vi "reward_behavior_michelle_visjitter_conswinAdapt_enticefx_TSLog_VF_fortraining_lightdetectionV2.vi"() -> ()   [LabVIEW 2019]
doc: "The myRIO Project template acquires acceleration data from the onboard accelerometer and displays the changes of acceleration values in a waveform chart."
uses:
  <vilib>/Analysis/Matrix/Datatypes/RealMatrix.ctl
  <vilib>/Utility/miscctls.llb/LVDateTimeRec.ctl
  <vilib>/myRIO/Instrument Drivers/Onboard IO/DIO/typedefs/DIO Reference.ctl
  <vilib>/myRIO/Common/Instrument Driver Framework/Utilities/typedefs/myRIO Generic Hardware Reference.ctl
  <vilib>/myRIO/Common/Instrument Driver Framework/Utilities/typedefs/Hardware Version Enum.ctl
  <vilib>/myRIO/Common/Instrument Driver Framework/Utilities/typedefs/myRIO v1.0 Reference.ctl
  <vilib>/myRIO/Common/Instrument Driver Framework/Utilities/typedefs/Generic FPGA Reference.ctl
  <vilib>/myRIO/Common/Instrument Driver Framework/myRIO v1.0/DIO/typedefs/DIO Channels List.ctl
  <vilib>/myRIO/Common/Instrument Driver Framework/myRIO v1.0/DIO/typedefs/DIO Channels Enum.ctl
  <vilib>/userdefined/High Color/nirio_resource_hc.ctl
  <vilib>/myRIO/Common/Instrument Driver Framework/myRIO v1.0/Encoder/typedefs/Encoder Signal Mode.ctl
  <vilib>/myRIO/Instrument Drivers/Onboard IO/Encoder/typedefs/Encoder Reference.ctl
  <vilib>/myRIO/Common/Instrument Driver Framework/myRIO v1.0/Encoder/typedefs/Encoder Channels Enum.ctl
  <vilib>/myRIO/Common/Instrument Driver Framework/myRIO v1.0/Encoder/typedefs/Encoder Configuration v1.0.ctl
  <vilib>/myRIO/Instrument Drivers/Onboard IO/AI/typedefs/AI Reference.ctl
  <vilib>/myRIO/Common/Instrument Driver Framework/myRIO v1.0/AI/typedefs/AI Channels List.ctl
  <vilib>/myRIO/Common/Instrument Driver Framework/myRIO v1.0/AI/typedefs/AI Channels Enum.ctl
  <vilib>/myRIO/Common/Instrument Driver Framework/Utilities/typedefs/Analog Scaling Constants List.ctl
  <vilib>/myRIO/Common/Instrument Driver Framework/Utilities/typedefs/Analog Scaling Constants.ctl
  <vilib>/myRIO/Instrument Drivers/Onboard IO/AO/typedefs/AO Reference.ctl
  <vilib>/myRIO/Common/Instrument Driver Framework/myRIO v1.0/AO/typedefs/AO Channels List.ctl
  <vilib>/myRIO/Common/Instrument Driver Framework/myRIO v1.0/AO/typedefs/AO Channels Enum.ctl
  <vilib>/myRIO/Common/Instrument Driver Framework/Utilities/vis/Is FPGA Ref Available.vi
  <vilib>/myRIO/Common/Instrument Driver Framework/myRIO v1.0/DIO/vis/myRIO v1.1 Open DIO.vi
  <vilib>/myRIO/Instrument Drivers/Onboard IO/DIO/vis/Write.vi
  <vilib>/myRIO/Common/Instrument Driver Framework/myRIO v1.0/Encoder/vis/myRIO v1.1 Open Encoder.vi
  <vilib>/myRIO/Instrument Drivers/Onboard IO/Encoder/vis/Read.vi
  <vilib>/myRIO/Common/Instrument Driver Framework/myRIO v1.0/AI/vis/myRIO v1.1 Open AI.vi
  <vilib>/myRIO/Instrument Drivers/Onboard IO/AI/vis/Read.vi
  <vilib>/myRIO/Common/Instrument Driver Framework/myRIO v1.0/AO/vis/myRIO v1.1 Open AO.vi
  <vilib>/myRIO/Instrument Drivers/Onboard IO/AO/vis/Write.vi
  <vilib>/myRIO/Instrument Drivers/Onboard IO/DIO/vis/Read.vi
  <vilib>/myRIO/Common/Instrument Driver Framework/Utilities/vis/Validate Channels.vi
  <vilib>/myRIO/Common/Instrument Driver Framework/myRIO v1.0/DIO/vis/myRIO v1.0 Reserve DIO.vi
  <vilib>/myRIO/Common/Instrument Driver Framework/myRIO v1.0/Encoder/vis/myRIO v1.0 Reserve Encoder.vi
  <vilib>/myRIO/Common/Instrument Driver Framework/myRIO v1.0/AI/vis/myRIO v1.0 Reserve AI.vi
  <vilib>/myRIO/Common/Instrument Driver Framework/myRIO v1.0/AO/vis/myRIO v1.0 Reserve AO.vi
  <vilib>/myRIO/Common/Instrument Driver Framework/myRIO v1.0/Resource Manager/vis/myRIO v1.0 Reserve Channel List.vi
  <vilib>/myRIO/Common/Instrument Driver Framework/myRIO v1.0/DIO/vis/myRIO v1.0 Build MUX Configuration DIO.vi
  <vilib>/myRIO/Common/Instrument Driver Framework/myRIO v1.0/Encoder/vis/myRIO v1.0 Build MUX Configuration Encoder.vi
  <vilib>/myRIO/Common/Instrument Driver Framework/myRIO v1.0/AI/vis/myRIO v1.0 Build MUX Configuration AI.vi
  <vilib>/myRIO/Common/Instrument Driver Framework/myRIO v1.0/AO/vis/myRIO v1.0 Build MUX Configuration AO.vi
  <vilib>/myRIO/Common/Instrument Driver Framework/myRIO v1.0/Resource Manager/vis/myRIO v1.0 Reserve Channel.vi
  <vilib>/myRIO/Common/Instrument Driver Framework/myRIO v1.0/Resource Manager/vis/myRIO v1.0 Unreserve Channel.vi
  <vilib>/myRIO/Common/Instrument Driver Framework/myRIO v1.0/Resource Manager/vis/myRIO v1.0 Create Configuration List.vi
  <vilib>/myRIO/Common/Instrument Driver Framework/myRIO v1.0/Resource Manager/vis/myRIO v1.0 Build Mutex Name.vi
  <vilib>/Utility/VariantDataType/GetNumericInfo.vi
  <vilib>/Utility/error.llb/Error Cluster From Error Code.vi
  <vilib>/myRIO/Common/Instrument Driver Framework/myRIO v1.0/myRIO v1.1 Open.vi
  <vilib>/myRIO/Common/Instrument Driver Framework/Utilities/vis/IO Manager.vi
  <vilib>/myRIO/Common/Instrument Driver Framework/Utilities/vis/Configuration Manager.vi
  <vilib>/myRIO/Common/Instrument Driver Framework/myRIO v1.0/Resource Manager/vis/myRIO v1.0 Configure IO.vi
  <vilib>/myRIO/Common/Instrument Driver Framework/myRIO v1.0/myRIO v1.0 Close.vi
  <vilib>/myRIO/Common/Instrument Driver Framework/myRIO v1.0/Encoder/vis/myRIO v1.0 Configure Encoder.vi
  <vilib>/myRIO/Common/Instrument Driver Framework/myRIO v1.0/Encoder/vis/myRIO v1.0 Read Encoder.vi
  <vilib>/myRIO/Common/Instrument Driver Framework/myRIO v1.0/DIO/vis/myRIO v1.0 Write DIO.vi
  <vilib>/myRIO/Common/Instrument Driver Framework/myRIO v1.0/DIO/vis/myRIO v1.0 Read DIO.vi
  <vilib>/myRIO/Common/Instrument Driver Framework/myRIO v1.0/AI/vis/myRIO v1.0 Get Scaling Constants AI.vi
  <vilib>/myRIO/Common/Instrument Driver Framework/myRIO v1.0/AI/vis/myRIO v1.0 Read AI.vi
  <vilib>/myRIO/Common/Instrument Driver Framework/myRIO v1.0/AO/vis/myRIO v1.0 Get Scaling Constants AO.vi
  <vilib>/myRIO/Common/Instrument Driver Framework/myRIO v1.0/AO/vis/myRIO v1.0 Write AO.vi
  <vilib>/myRIO/Express VI/Onboard IO/Encoder/Encoder Express VI.xnode
  <vilib>/myRIO/Instrument Drivers/Onboard IO/Encoder/vis/myRIO Encoder Open.xnode
  <vilib>/myRIO/Common/Instrument Driver Framework/myRIO v1.0/Encoder/typedefs/Encoder Count Direction Enum.ctl
  <vilib>/myRIO/Express VI/Onboard IO/DO/DO Express VI.xnode
  <vilib>/myRIO/Instrument Drivers/Onboard IO/DIO/vis/myRIO DIO Open.xnode
  <vilib>/myRIO/Express VI/Onboard IO/DI/DI Express VI.xnode
  <vilib>/myRIO/Express VI/Onboard IO/AI/AI Express VI.xnode
  <vilib>/myRIO/Instrument Drivers/Onboard IO/AI/vis/myRIO AI Open.xnode
  <vilib>/myRIO/Express VI/Onboard IO/AO/AO Express VI.xnode
  <vilib>/myRIO/Instrument Drivers/Onboard IO/AO/vis/myRIO AO Open.xnode
  <vilib>/myRIO/Instrument Drivers/Onboard IO/Encoder/Encoder.lvlib
  <vilib>/myRIO/Instrument Drivers/Onboard IO/DIO/DIO.lvlib
  <vilib>/myRIO/Instrument Drivers/Onboard IO/AI/AI.lvlib
  <vilib>/myRIO/Instrument Drivers/Onboard IO/AO/AO.lvlib
  <vilib>/Analysis/Matrix/NI_Matrix.lvlib
panel:
  out "StartTime":dbl
  out "TimeStampTime":dbl
  out "initiatedlag":dbl
  out "NeedLag":bool=TRUE
  out "date time rec":T1
  out "InitiationLag":i32
  out "LightTrig":bool=TRUE
  out "LightAvg":dbl=0.15
  out "LimitCalc":dbl
  out "LightLimit":dbl
  out "LightTS":dbl[][](array[numeric])
  out "LightDerivPlot":dbl[](graph)
  out "LightDeriv":dbl
  out "LightOn":bool=TRUE
  out "Light":dbl
  out "Lightplot":dbl[](graph)
  out "LightArray":dbl[](array[numeric])
  out "AutoEnticeLimit":i32=1000
  out "GetVidFrame":i32
  out "VidTS":dbl[][](array[numeric])
  out "EntTS":dbl[][](array[numeric])
  out "TimeLag":dbl
  out "Lag2":dbl
  out "TestTime":dbl
  out "RewTS":dbl[][](array[numeric])
  out "ConsTS":dbl[][](array[numeric])
  out "LickTS":dbl[][](array[numeric])
  out "ContrastChoice":dbl
  out "Its":i32
  out "BurstCriteria":dbl
  out "LickBurst 2":bool
  out "LickBurst":bool
  out "Enticements":i32
  in  "Entice":bool
  out "Misses":i32
  out "GoAhead":bool
  out "TimeOutDuration":i32
  out "ActiveTime":dbl
  out "ConsumptionGo":bool=TRUE
  out "Consumption_Period":i32
  out "Watch_Display":bool=TRUE
  in  "Give reward":bool
  out "Timings":dbl[](array[numeric])
  out "ISI":dbl
  out "ISI start time":dbl
  out "Time_out":bool=TRUE
  out "Time since lick":dbl
  out "Time of last lick":dbl
  out "Rewarded trials":dbl[](array[numeric])
  out "Rewards":u16
  out "Active Trial":bool
  out "Array temp2":T2
  out "Stimuli Loaded":bool
  out "Stim_ID":dbl[](array[numeric])
  out "Reward_mat":dbl[](array[numeric])
  out "Reward":bool=TRUE
  out "Frame clock":i32
  out "Licks":u32
  out "Lick":bool
  out "Time":dbl
  out "Stop":bool
  in  "Frames to collect":u32
  out "Overflow?":bool
  out "Counter Value":i32
  out "Velocity":dbl
  out "Velocity Plot":dbl[](graph)
  out "Velocity array":dbl[](array[numeric])
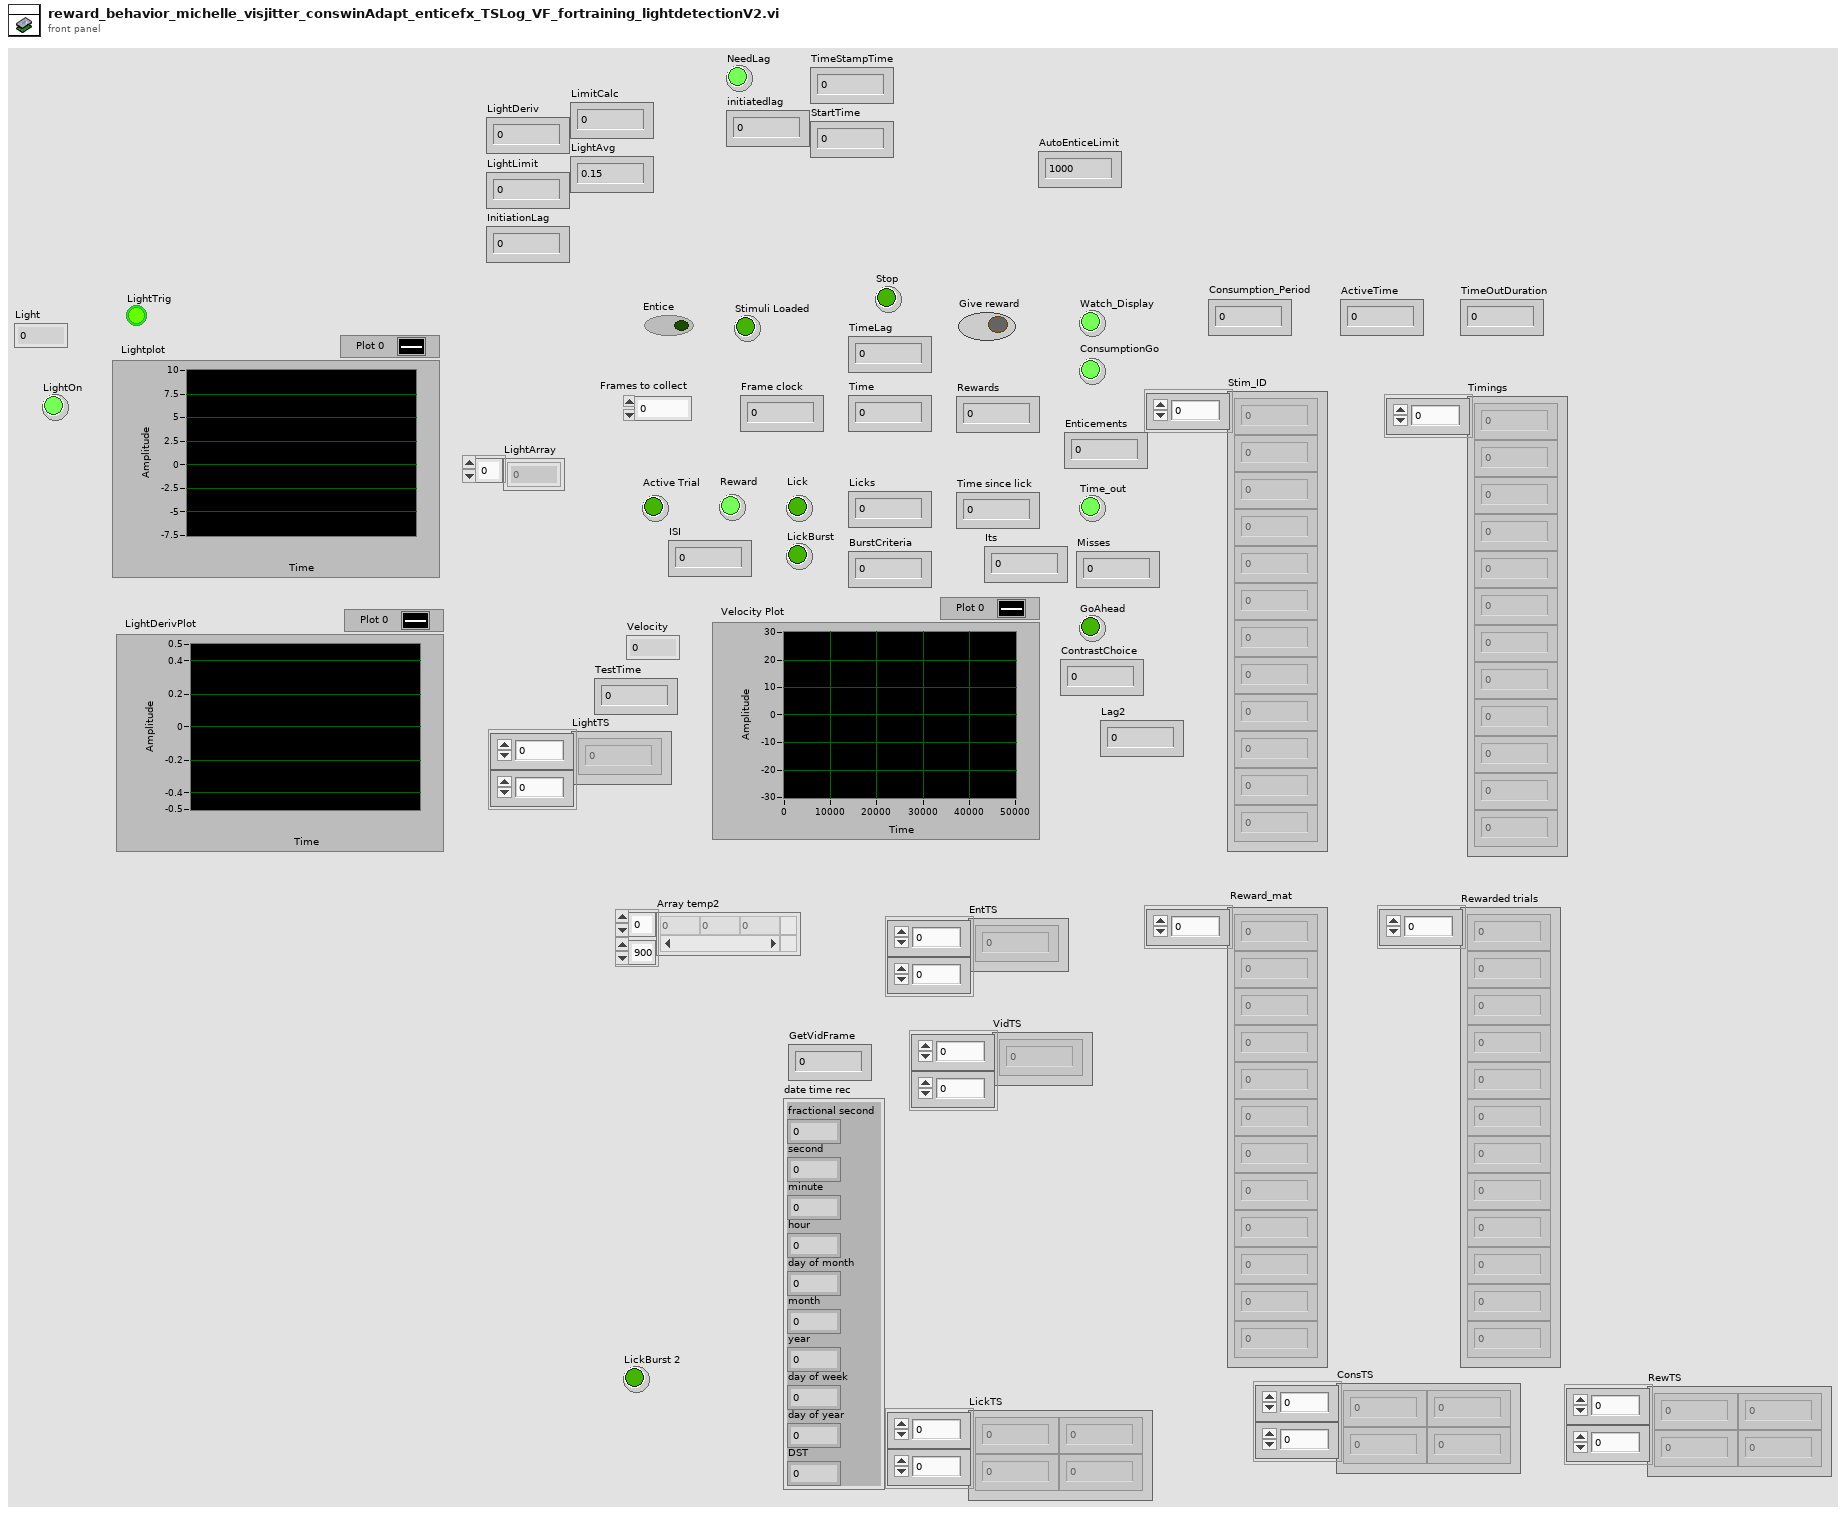
[diagram p1: front panel]
types:
  T1 = typedef "LVDateTimeRec.ctl" = cluster{"fractional second":dbl, "second":i32, "minute":i32, "hour":i32, "day of month":i32, "month":i32, "year":i32, "day of week":i32, "day of year":i32, "DST":i32}
  T2 = typedef "NI_Matrix.lvlib/RealMatrix.ctl" = dbl[][]
  T3 = typedef "DIO.lvlib/DIO Reference.ctl" = cluster{"myRIO Reference":T4, "DIO Channels List":T8}
  T4 = typedef "myRIO Generic Hardware Reference.ctl" = cluster{"myRIO Model":T5, "myRIO Hardware Reference":T6}
  T5 = typedef "Hardware Version Enum.ctl" = enum16{"Unknown", "myRIO-1900", "myRIO-1950", "roboRIO", "NI ELVIS RIO CM", "ELVIS III"}
  T6 = typedef "myRIO v1.0 Reference.ctl" = cluster{"Generic FPGA Reference":T7, "Allow multiple opens":bool}
  T7 = typedef "Generic FPGA Reference.ctl" = refnum<k20>
  T8 = typedef "DIO Channels List.ctl" = T9[]
  T9 = typedef "DIO Channels Enum.ctl" = enum16{"Not Connected", "C/DIO0", "C/DIO1", "C/DIO2", "C/DIO3", "C/DIO4", "C/DIO5", "C/DIO6", "C/DIO7", "A/DIO0", "A/DIO1", "A/DIO2", "A/DIO3", "A/DIO4", "A/DIO5", "A/DIO6", "A/DIO7", "A/DIO8", "A/DIO9", "A/DIO10", "A/DIO11", "A/DIO12", "A/DIO13", "A/DIO14", "A/DIO15", "A/DIO16", "A/DIO17", "A/DIO18", "A/DIO19", "B/DIO0", "B/DIO1", "B/DIO2", "B/DIO3", "B/DIO4", "B/DIO5", "B/DIO6", "B/DIO7", "B/DIO8", "B/DIO9", "B/DIO10", "B/DIO11", "B/DIO12", "B/DIO13", "B/DIO14", "B/DIO15", "B/DIO16", "B/DIO17", "B/DIO18", "B/DIO19", "LED0", "LED1", "LED2", "LED3", "Button0", "DIO/DIO0", "DIO/DIO1", "DIO/DIO2", "DIO/DIO3", "DIO/DIO4", "DIO/DIO5", "DIO/DIO6", "DIO/DIO7", "DIO/DIO8", "DIO/DIO9", "SPI/CS0", "SPI/CS1", "SPI/CS2", "SPI/CS3", "LED RADIO (Green)", "LED RADIO (Red)", "LED COMM (Green)", "LED COMM (Red)", "LED MODE (Green)", "LED MODE (Red)"}
  T10 = typedef "nirio_resource_hc.ctl" = tag
  T11 = typedef "Encoder.lvlib/Encoder Reference.ctl" = cluster{"myRIO Reference":T4, "Encoder Channels Enum":T12}
  T12 = typedef "Encoder Channels Enum.ctl" = enum16{"Not Connected", "C/ENC0", "C/ENC1", "A/ENC", "A/ENC0", "A/ENC1", "A/ENC2", "A/ENC3", "A/ENC4", "A/ENC5", "A/ENC6", "A/ENC7", "A/ENC8", "A/ENC9", "B/ENC", "B/ENC0", "B/ENC1", "B/ENC2", "B/ENC3", "B/ENC4", "B/ENC5", "B/ENC6", "B/ENC7", "B/ENC8", "B/ENC9", "DIO/ENC0", "DIO/ENC1", "DIO/ENC2", "DIO/ENC3", "DIO/ENC4"}
  T13 = typedef "Encoder Signal Mode.ctl" = enum16{"Quadrature phase signal", "Step and direction signal"}
  T14 = typedef "AO.lvlib/AO Reference.ctl" = cluster{"myRIO Reference":T4, "AO Channel List":T15, "AO Scaling Constant List":T17}
  T15 = typedef "AO Channels List.ctl" = T16[]
  T16 = typedef "AO Channels Enum.ctl" = enum16{"Not Connected", "AudioOut/Left", "AudioOut/Right", "C/AO0", "C/AO1", "A/AO0", "A/AO1", "B/AO0", "B/AO1"}
  T17 = typedef "Analog Scaling Constants List.ctl" = T18[]
  T18 = typedef "Analog Scaling Constants.ctl" = cluster{"LSB Weight (Volts)":dbl, "Offset (Volts)":dbl, "Signed?":bool}
  T19 = typedef "AI.lvlib/AI Reference.ctl" = cluster{"myRIO Reference":T4, "AI Channels List":T20, "AI Scaling Constants List":T17}
  T20 = typedef "AI Channels List.ctl" = T21[]
  T21 = typedef "AI Channels Enum.ctl" = enum16{"Not Connected", "AudioIn/Left", "AudioIn/Right", "C/AI0", "C/AI1", "A/AI0", "A/AI1", "A/AI2", "A/AI3", "A/AI4", "A/AI5", "A/AI6", "A/AI7", "B/AI0", "B/AI1", "B/AI2", "B/AI3", "B/AI4", "B/AI5", "B/AI6", "B/AI7", "AI/AI0", "AI/AI1", "AI/AI2", "AI/AI3", "A/AI0 (DIFF)", "A/AI1 (DIFF)", "A/AI2 (DIFF)", "A/AI3 (DIFF)", "B/AI0 (DIFF)", "B/AI1 (DIFF)", "B/AI2 (DIFF)", "B/AI3 (DIFF)"}
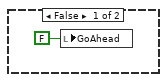
[diagram p8: hidden frame]
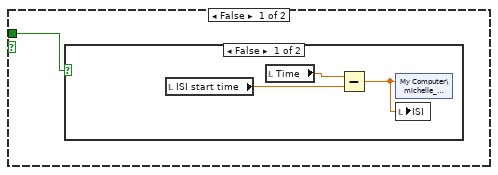
[diagram p14: hidden frame]
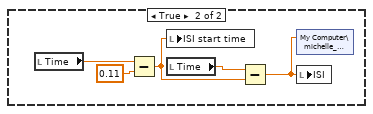
[diagram p15: hidden frame]
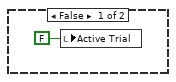
[diagram p16: hidden frame]
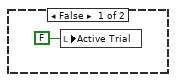
[diagram p17: hidden frame]
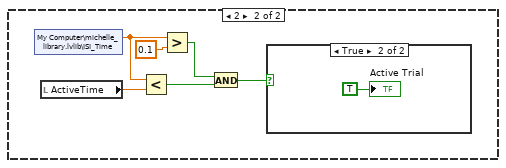
[diagram p18: hidden frame]
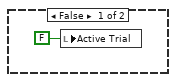
[diagram p19: hidden frame]
diagram:
  n1 = flat-sequence {
    frame #0 {
      w8 = 0.0
      w30 = FALSE ("Time_out")
      n2 = flat-sequence {
        frame #0 {
          w42 = TRUE
          n3 = xnode "DisplayOn 5"("C/DIO2 (DIO2)"=w42) -> ()  [unwired: 1 in, 1 out]
          n4 = xnode "DisplayOn 6"("C/DIO1 (DIO1)"=w42) -> ()  [unwired: 1 in, 1 out]
          n5 = xnode "BootUp"("C/DIO3 (DIO3)"=w42) -> ()  [unwired: 1 in, 1 out]
        }
        frame #1 {
          n6 = Wait (ms)(milliseconds to wait=210) -> ()  [unwired: 1 out]
        }
        frame #2 {
          w149 = FALSE
          n7 = xnode "BootUp 3"("C/DIO2 (DIO2)"=w149) -> ()  [unwired: 1 in, 1 out]
          n8 = xnode "BootUp 5"("C/DIO3 (DIO3)"=w149) -> ()  [unwired: 1 in, 1 out]
          n9 = xnode "BootUp 4"("C/DIO1 (DIO1)"=w149) -> ()  [unwired: 1 in, 1 out]
        }
      }
      n10 = Get Date/Time In Seconds() -> (seconds since 1Jan1904=w2:timestamp)
      n11 = To Double Precision Float(number=w2) -> (double precision float=→"StartTime":dbl)
      n12 = Get Date/Time In Seconds() -> (seconds since 1Jan1904=w14:timestamp)
      n13 = Initialize Array(0.0, 1, 3) -> (w11:dbl[][])
      "LickTS" <- w11
      "ConsTS" <- w11
      "RewTS" <- w11
      "EntTS" <- w11
      "VidTS" <- w11
      "LightTS" <- w11
      n14 = local write "Licks"(u32 0 ("Licks")) -> ()
      n15 = local write "Velocity"(0.0 ("Velocity")) -> ()
      n16 = shared-variable "My Computer\\michelle_library.lvlib\\GlobalReward"(0.0) -> ()  [unwired: 1 in, 1 out]
      n17 = local write "Rewards"(u16 0 ("Rewards")) -> ()
      n18 = shared-variable "My Computer\\michelle_library.lvlib\\Display"(FALSE ("Display")) -> ()  [unwired: 1 in, 1 out]
      n19 = local write "Lick"(FALSE ("Lick")) -> ()
      n20 = shared-variable "My Computer\\michelle_library.lvlib\\Stim_loaded"(FALSE ("Stim_loaded")) -> ()  [unwired: 1 in, 1 out]
      n21 = shared-variable "My Computer\\michelle_library.lvlib\\Stop"(FALSE ("Stop")) -> ()  [unwired: 1 in, 1 out]
      n22 = local write "Reward"(FALSE ("Give reward")) -> ()
      n23 = local write "ConsumptionGo"(FALSE ("ConsumptionGo")) -> ()
      n24 = local write "Watch_Display"(FALSE ("Watch_Display")) -> ()
      n25 = xnode "Encoder 2"("Reset Counter"=TRUE) -> ()  [unwired: 1 in, 4 out]
      n26 = xnode "Velocity encoder 2"("Reset Counter"=TRUE) -> ()  [unwired: 1 in, 4 out]
      n27 = Wait (ms)(milliseconds to wait=u32 10) -> ()  [unwired: 1 out]
      n28 = local write "Time_out"(w30) -> ()
      n29 = shared-variable "My Computer\\michelle_library.lvlib\\Timeout"(w30) -> ()  [unwired: 1 in, 1 out]
      n30 = To Double Precision Float(number=w14) -> (double precision float=→"TestTime":dbl)
      n31 = shared-variable "My Computer\\michelle_library.lvlib\\TSLog_Behavior"(w11) -> ()  [unwired: 1 in, 1 out]
      n32 = local write "Frame clock"(u32 0 ("Frames")) -> ()
      "Consumption_Period" <- 2500
      "ActiveTime" <- 0.6
      "TimeOutDuration" <- 3000
      "GoAhead" <- FALSE
      "Misses" <- 0
      "Enticements" <- 0
      "LickBurst" <- FALSE
      "BurstCriteria" <- 0.5
      "Its" <- 0
      "GetVidFrame" <- 1
      "AutoEnticeLimit" <- 3
      "LightDeriv" <- w8
      "LightLimit" <- 100.0
      "LimitCalc" <- w8
      "InitiationLag" <- 0
      "NeedLag" <- TRUE
      "initiatedlag" <- 0.0
      "TimeStampTime" <- 0.0
    }
    frame #1 {
      n33 = while {
        stop <- w714 stop-if-true
        n34 = local read "TimeStampTime"() -> (w703:dbl)
        n35 = local read "Time"() -> (w704:dbl)
        n36 = local read "Velocity"() -> (w718:dbl)
        n37 = local read "ConsumptionGo"() -> (w712:bool)
        n38 = local read "Give reward"() -> (w711:bool)
        n39 = local read "LickBurst"() -> (w708:bool)
        n40 = local read "Reward"() -> (w719:bool)
        n41 = local read "Lick"() -> (w720:bool)
        n42 = Boolean To (0,1)(Boolean=w719) -> (0, 1=w717:i16)
        n43 = Boolean To (0,1)(Boolean=w720) -> (0, 1=w716:i16)
        n44 = Boolean To (0,1)(Boolean=w712) -> (0, 1=w710:i16)
        n45 = Boolean To (0,1)(Boolean=w711) -> (0, 1=w709:i16)
        n46 = Boolean To (0,1)(Boolean=w708) -> (0, 1=w707:i16)
        n47 = local read "Light"() -> (w706:dbl)
        n48 = local read "LightDeriv"() -> (w705:dbl)
        n49 = Build Array(w704, w703, w718, w717, w716, w710, w709, w707, w706, w705) -> (w713:T2)
        "Array temp2" <- w713
        n50 = shared-variable "My Computer\\michelle_library.lvlib\\Array temp2"(w713) -> ()  [unwired: 1 in, 1 out]
        n51 = local read "Stop"() -> (w714:bool)
        n52 = Wait (ms)(milliseconds to wait=u32 1) -> ()  [unwired: 1 out]
      }
      n53 = Tick Count (ms)() -> (millisecond timer value=w347:u32)
      n54 = flat-sequence {
        frame #0 {
          n55 = while {
            stop <- w1033 stop-if-true
            n56 = xnode "Encoder"() -> ("Counter Value"=w1036:i32)  [unwired: 2 in, 3 out]
            n57 = Multiply(x=w1036, y=-1) -> (x*y=w1032:i32)
            "Frame clock" <- w1032
            n58 = shared-variable "My Computer\\michelle_library.lvlib\\Frame_clock"(w1032) -> ()  [unwired: 1 in, 1 out]
            n59 = Equal?(x=w1032, y="Frames to collect") -> (x = y?=w1033:bool)
            "Stop" <- w1033
            n60 = Wait (ms)(milliseconds to wait=u32 1) -> ()  [unwired: 1 out]
          }
        }
        frame #1 {
          n61 = local read "Stop"() -> (w1084:bool)
          n62 = shared-variable "My Computer\\michelle_library.lvlib\\Stop"(w1084) -> ()  [unwired: 1 in, 1 out]
        }
      }
      n63 = while {
        shift-right: [w1171] -> _
        shift-left: _ -> [w1172]
        shift-right: [w1163] -> _
        shift-left: _ -> [w1162]
        stop <- w1161 stop-if-true
        n64 = xnode "Encoder"() -> ("Counter Value"=w1171:i32, "Overflow?"=→"Overflow?":bool)  [unwired: 2 in, 2 out]
        "Counter Value" <- w1171
        n65 = Wait (ms)(milliseconds to wait=u32 1) -> ()  [unwired: 1 out]
        n66 = Subtract(x=w1171, y=w1172) -> (x-y=w1164:i32)
        n67 = Divide(x=w1164, y=1200.0 ("600")) -> (x/y=w1169:dbl)
        n68 = Multiply(x=w1169, y=34.5) -> (x*y=w1167:dbl)
        n69 = Multiply(x=20.0, y=w1167) -> (x*y=w1165:dbl)
        "Velocity" <- w1165
        n70 = Build Array (concatenate)(w1162, w1165) -> (w1163:dbl[])
        "Velocity Plot" <- w1163
        "Velocity array" <- w1163
        n71 = local read "Stop"() -> (w1161:bool)
      }
      n72 = while {
        shift-right: [w1097] -> _
        shift-left: _ -> [w1096]
        shift-right: [w1091] -> _
        shift-left: _ -> [w1094]
        shift-right: [w1085] -> _
        shift-left: _ -> [w1086]
        stop <- w1095 stop-if-true
        n73 = local read "LickBurst"() -> (w1088:bool)
        n74 = Wait (ms)(milliseconds to wait=u32 10) -> ()  [unwired: 1 out]
        n75 = xnode "Lick sensor"() -> ("C/DIO1 (DIO1)"=w1091:bool)  [unwired: 1 in, 1 out]
        "Lick" <- w1091
        n76 = Not(x=w1088) -> (.not. x?=w1087:bool)
        n77 = Not(x=w1094) -> (.not. x?=w1093:bool)
        n78 = local read "Lick"() -> (w1089:bool)
        n79 = And(x=w1087, y=w1089) -> (x .and. y?=w1090:bool)
        n80 = And(x=w1093, y=w1091) -> (x .and. y?=w1092:bool)
        n81 = case shown="True" w1090 {
          frame False {
          }
          frame True {
            n82 = local write "LickBurst"(TRUE) -> ()
          }
        }
        n83 = case shown="True" w1092 {
          tunnel: [w1104 w1114] -> w1097
          tunnel: w1096 -> [w1104 w1113]
          tunnel: w1086 -> [w1100 w1105]
          tunnel: [w1100 w1107] -> w1085
          frame False {
            n84 = local read "Time of last lick"() -> (w1102:dbl)
            n85 = local read "Time"() -> (w1103:dbl)
            n86 = Subtract(x=w1103, y=w1102) -> (x-y=w1101:dbl)
            n87 = shared-variable "My Computer\\michelle_library.lvlib\\Time_since_lick"(w1101) -> ()  [unwired: 1 in, 1 out]
            n88 = local write "Time since lick"(w1101) -> ()
          }
          frame True {
            n89 = local read "Time"() -> (w1110:dbl)
            n90 = local read "Lick"() -> (w1106:bool)
            n91 = Increment(x=w1113) -> (x+1=w1114:u32)
            "Licks" <- w1114
            n92 = case shown="True" w1106 {
              tunnel: w1105 -> [w1115 w1121]
              tunnel: [w1115 w1120] -> w1107
              frame False {
              }
              frame True {
                n93 = shared-variable "My Computer\\michelle_library.lvlib\\Frame_clock"() -> (w1116:u32)  [unwired: 1 in, 1 out]
                n94 = Get Date/Time In Seconds() -> (seconds since 1Jan1904=w1123:timestamp)
                n95 = local read "TestTime"() -> (w1118:dbl)
                n96 = To Double Precision Float(number=w1123) -> (double precision float=w1119:dbl)
                n97 = shared-variable "My Computer\\michelle_library.lvlib\\GlobalTime"() -> (w1117:dbl)  [unwired: 1 in, 1 out]
                n98 = Subtract(x=w1119, y=w1118) -> (x-y=w1124:dbl)
                n99 = Build Array(441, w1124, w1117, w1116) -> (w1125:T2)
                n100 = Build Array (concatenate) ("Build Matrix")(w1121, w1125) -> (w1120:T2)
                n101 = local write "LickTS"(w1120) -> ()
              }
            }
            n102 = Subtract(x=w1110, y=0.11) -> (x-y=w1108:dbl)
            "Time of last lick" <- w1108
            n103 = local read "Time"() -> (w1112:dbl)
            n104 = Subtract(x=w1112, y=w1108) -> (x-y=w1111:dbl)
            "Time since lick" <- w1111
            n105 = shared-variable "My Computer\\michelle_library.lvlib\\Time_since_lick"(w1111) -> ()  [unwired: 1 in, 1 out]
          }
        }
        n106 = local read "Stop"() -> (w1095:bool)
      }
      n107 = while {
        stop <- w499 stop-if-true
        n108 = local read "LickBurst"() -> (w497:bool)
        n109 = Wait (ms)(milliseconds to wait=u32 10) -> ()  [unwired: 1 out]
        n110 = case shown="True" w497 {
          frame False {
          }
          frame True {
            n111 = flat-sequence {
              frame #0 {
                n112 = while {
                  stop <- w502 stop-if-true
                  n113 = local read "Time since lick"() -> (w503:dbl)
                  n114 = local read "BurstCriteria"() -> (w504:dbl)
                  n115 = Subtract(x=w503, y=w504) -> (x-y=w500:dbl)
                  n116 = Greater?(x=w500, y=0.0) -> (0:w502:bool)
                }
              }
              frame #1 {
                n117 = local write "LickBurst"(FALSE) -> ()
              }
            }
          }
        }
        n118 = shared-variable "My Computer\\michelle_library.lvlib\\Stop"() -> (w499:bool)  [unwired: 1 in, 1 out]
      }
      n119 = while {
        tunnel: w347 -> [w1237]
        stop <- w1235 stop-if-true
        n120 = local read "StartTime"() -> (w1221:dbl)
        n121 = local read "EntTS"() -> (w1228:dbl[][])
        n122 = local read "VidTS"() -> (w1227:dbl[][])
        n123 = Tick Count (ms)() -> (millisecond timer value=w1238:u32)
        n124 = Wait (ms)(milliseconds to wait=u32 1) -> ()  [unwired: 1 out]
        n125 = local read "ConsTS"() -> (w1231:dbl[][])
        n126 = Get Date/Time In Seconds() -> (seconds since 1Jan1904=w1222:timestamp)
        n127 = Subtract(x=w1238, y=w1237) -> (x-y=w1234:u32)
        n128 = local read "LightTS"() -> (w1226:dbl[][])
        n129 = local read "RewTS"() -> (w1230:dbl[][])
        n130 = local read "LickTS"() -> (w1232:dbl[][])
        n131 = To Double Precision Float(number=w1222) -> (double precision float=w1224:dbl)
        n132 = Divide(x=w1234, y=u32 1000) -> (x/y=→"Time":dbl)
        n133 = Build Array (concatenate) ("Build Matrix")(w1232, w1231, w1230, w1228, w1227, w1226) -> (w1229:T2)
        n134 = Subtract(x=w1224, y=w1221) -> (x-y=w1223:dbl)
        n135 = local write "TimeStampTime"(w1223) -> ()
        n136 = shared-variable "My Computer\\michelle_library.lvlib\\TSLog_Behavior"(w1229) -> ()  [unwired: 1 in, 1 out]
        n137 = local read "Stop"() -> (w1235:bool)
      }
      n138 = while {
        stop <- w487 stop-if-true
        n139 = local read "NeedLag"() -> (w484:bool)
        n140 = shared-variable "My Computer\\michelle_library.lvlib\\Stim_loaded"() -> (w485:bool)  [unwired: 1 in, 1 out]
        n141 = Wait (ms)(milliseconds to wait=u32 1) -> ()  [unwired: 1 out]
        n142 = shared-variable "My Computer\\michelle_library.lvlib\\Stim_loaded"() -> (w488:bool)  [unwired: 1 in, 1 out]
        n143 = And(x=w485, y=w484) -> (x .and. y?=w483:bool)
        n144 = case shown="True" w488 {
          frame False {
          }
          frame True {
            n145 = shared-variable "My Computer\\michelle_library.lvlib\\GlobalTime"() -> (w494:dbl)  [unwired: 1 in, 1 out]
            n146 = local read "Time"() -> (w495:dbl)
            n147 = Subtract(x=w494, y=w495) -> (x-y=→"TimeLag":dbl)
          }
        }
        n148 = case shown="True" w483 {
          frame False {
          }
          frame True {
            n149 = shared-variable "My Computer\\michelle_library.lvlib\\InitiatedLag"() -> (w489:dbl)  [unwired: 1 in, 1 out]
            n150 = Get Date/Time In Seconds() -> (seconds since 1Jan1904=w491:timestamp)
            n151 = To Double Precision Float(number=w491) -> (double precision float=w490:dbl)
            n152 = Subtract(x=w490, y=w489) -> (x-y=w492:dbl)
            n153 = local write "initiatedlag"(w492) -> ()
            n154 = local write "NeedLag"(FALSE) -> ()
          }
        }
        n155 = local read "Stop"() -> (w487:bool)
      }
      n156 = while {
        shift-right: [w514] -> _
        shift-left: _ -> [w515]
        stop <- w525 stop-if-true
        n157 = local read "AutoEnticeLimit"() -> (w506:i32)
        n158 = local read "Misses"() -> (w507:i32)
        n159 = shared-variable "My Computer\\michelle_library.lvlib\\EnticeLimiter"() -> (w513:dbl)  [unwired: 1 in, 1 out]
        n160 = shared-variable "My Computer\\michelle_library.lvlib\\Display"() -> (w524:bool)  [unwired: 1 in, 1 out]
        n161 = shared-variable "My Computer\\michelle_library.lvlib\\Display"() -> (w522:bool)  [unwired: 1 in, 1 out]
        n162 = shared-variable "My Computer\\michelle_library.lvlib\\ContrastChoice"() -> (w509:dbl)  [unwired: 1 in, 1 out]
        n163 = Wait (ms)(milliseconds to wait=35) -> ()  [unwired: 1 out]
        n164 = shared-variable "My Computer\\michelle_library.lvlib\\ContrastChoice"() -> (w518:dbl)  [unwired: 1 in, 1 out]
        n165 = shared-variable "My Computer\\michelle_library.lvlib\\ContrastChoice"() -> (→"ContrastChoice":dbl)  [unwired: 1 in, 1 out]
        n166 = Greater?(x=w507, y=w506) -> (0:w523:bool)
        n167 = case shown="True" w524 {
          frame False {
            n168 = local write "GoAhead"(FALSE) -> ()
          }
          frame True {
            n169 = flat-sequence {
              frame #0 {
                n170 = xnode "Reward"("C/DIO2 (DIO2)"=TRUE) -> ()  [unwired: 1 in, 1 out]
                n171 = local write "GoAhead"(TRUE) -> ()
              }
              frame #1 {
                n172 = while {
                  stop <- w608 continue-if-true
                  n173 = shared-variable "My Computer\\michelle_library.lvlib\\Display"() -> (w608:bool)  [unwired: 1 in, 1 out]
                  n174 = Wait (ms)(milliseconds to wait=1) -> ()  [unwired: 1 out]
                }
              }
              frame #2 {
                n175 = xnode "DisplayOn 2"("C/DIO2 (DIO2)"=FALSE) -> ()  [unwired: 1 in, 1 out]
                n176 = local read "GoAhead"() -> (w610:bool)
                n177 = case shown="True" w610 {
                  frame False {
                  }
                  frame True {
                    n178 = local read "Misses"() -> (w649:i32)
                    n179 = local write "GoAhead"(FALSE) -> ()
                    n180 = Add(x=w649, y=1) -> (x+y=w647:i32)
                    n181 = local write "Misses"(w647) -> ()
                  }
                }
              }
            }
          }
        }
        n182 = local read "Entice"() -> (w521:bool)
        n183 = case shown="True" w523 {
          frame False {
          }
          frame True {
            n184 = local write "Entice"(TRUE) -> ()
          }
        }
        n185 = And(x=w522, y=w521) -> (x .and. y?=w519:bool)
        n186 = Greater?(x=w509, y=0.02) -> (0:w510:bool)
        n187 = Greater?(x=w518, y=w513) -> (0:w511:bool)
        n188 = Or(x=w511, y=w510) -> (x .or. y?=w512:bool)
        n189 = And(x=w519, y=w512) -> (x .and. y?=w517:bool)
        n190 = case shown="True" w517 {
          tunnel: w515 -> [w526 w530]
          tunnel: [w526 w527] -> w514
          frame False {
          }
          frame True {
            n191 = flat-sequence {
              tunnel: w530 -> [w538]
              tunnel: [w537] -> w529
              tunnel: w529 -> [w548]
              tunnel: [w548] -> w528
              tunnel: w528 -> [w556]
              tunnel: [w555] -> w527
              frame #0 {
                n192 = shared-variable "My Computer\\michelle_library.lvlib\\Frame_clock"() -> (w536:u32)  [unwired: 1 in, 1 out]
                n193 = Get Date/Time In Seconds() -> (seconds since 1Jan1904=w545:timestamp)
                n194 = local read "TestTime"() -> (w540:dbl)
                n195 = shared-variable "My Computer\\michelle_library.lvlib\\GlobalReward"() -> (w547:dbl)  [unwired: 1 in, 1 out]
                n196 = To Double Precision Float(number=w545) -> (double precision float=w544:dbl)
                n197 = shared-variable "My Computer\\michelle_library.lvlib\\GlobalTime"() -> (w539:dbl)  [unwired: 1 in, 1 out]
                n198 = Get Date/Time In Seconds() -> (seconds since 1Jan1904=w534:timestamp)
                n199 = To Double Precision Float(number=w534) -> (double precision float=w531:dbl)
                n200 = Subtract(x=w544, y=w540) -> (x-y=w543:dbl)
                n201 = Increment(x=w547) -> (x+1=w546:dbl)
                n202 = shared-variable "My Computer\\michelle_library.lvlib\\GlobalReward"(w546) -> ()  [unwired: 1 in, 1 out]
                n203 = local read "initiatedlag"() -> (w533:dbl)
                n204 = Subtract(x=w531, y=w533) -> (x-y=w532:dbl)
                n205 = Build Array(661, w543, w539, w536, w532) -> (w542:T2)
                n206 = Build Array (concatenate) ("Build Matrix")(w538, w542) -> (w537:T2)
                n207 = Seconds To Date/Time(time stamp (now)=w534) -> (date time rec=→"date time rec":T1)  [unwired: 1 in]
                n208 = local write "EntTS"(w537) -> ()
              }
              frame #1 {
                n209 = Wait (ms)(milliseconds to wait=200) -> ()  [unwired: 1 out]
              }
              frame #2 {
                n210 = shared-variable "My Computer\\michelle_library.lvlib\\Frame_clock"() -> (w554:u32)  [unwired: 1 in, 1 out]
                n211 = Get Date/Time In Seconds() -> (seconds since 1Jan1904=w563:timestamp)
                n212 = local read "Enticements"() -> (w565:i32)
                n213 = local write "Entice"(FALSE) -> ()
                n214 = local write "Give reward"(TRUE) -> ()
                n215 = local read "TestTime"() -> (w557:dbl)
                n216 = To Double Precision Float(number=w563) -> (double precision float=w562:dbl)
                n217 = shared-variable "My Computer\\michelle_library.lvlib\\GlobalTime"() -> (w558:dbl)  [unwired: 1 in, 1 out]
                n218 = Subtract(x=w562, y=w557) -> (x-y=w561:dbl)
                n219 = Increment(x=w565) -> (x+1=w564:i32)
                n220 = Get Date/Time In Seconds() -> (seconds since 1Jan1904=w553:timestamp)
                n221 = local write "Enticements"(w564) -> ()
                n222 = To Double Precision Float(number=w553) -> (double precision float=w552:dbl)
                n223 = local read "initiatedlag"() -> (w550:dbl)
                n224 = Subtract(x=w552, y=w550) -> (x-y=w551:dbl)
                n225 = Build Array(662, w561, w558, w554, w551) -> (w560:T2)
                n226 = Build Array (concatenate) ("Build Matrix")(w556, w560) -> (w555:T2)
                n227 = local write "EntTS"(w555) -> ()
              }
            }
          }
        }
        n228 = shared-variable "My Computer\\michelle_library.lvlib\\Stop"() -> (w525:bool)  [unwired: 1 in, 1 out]
      }
      n229 = while {
        stop <- w349 stop-if-true
        n230 = flat-sequence {
          frame #0 {
            n231 = local read "Light"() -> (w350:dbl)
            n232 = local write "LimitCalc"(w350) -> ()
          }
          frame #1 {
            n233 = Wait (ms)(milliseconds to wait=u32 50) -> ()  [unwired: 1 out]
          }
          frame #2 {
            n234 = local read "LimitCalc"() -> (w353:dbl)
            n235 = local read "Light"() -> (w354:dbl)
            n236 = Add(x=w353, y=w354) -> (x+y=w352:dbl)
            n237 = local write "LimitCalc"(w352) -> ()
          }
          frame #3 {
            n238 = Wait (ms)(milliseconds to wait=u32 50) -> ()  [unwired: 1 out]
          }
          frame #4 {
            n239 = local read "LimitCalc"() -> (w356:dbl)
            n240 = local read "Light"() -> (w357:dbl)
            n241 = Add(x=w356, y=w357) -> (x+y=w358:dbl)
            n242 = local write "LimitCalc"(w358) -> ()
          }
          frame #5 {
            n243 = Wait (ms)(milliseconds to wait=u32 50) -> ()  [unwired: 1 out]
          }
          frame #6 {
            n244 = local read "LimitCalc"() -> (w361:dbl)
            n245 = local read "Light"() -> (w362:dbl)
            n246 = Add(x=w361, y=w362) -> (x+y=w360:dbl)
            n247 = local write "LimitCalc"(w360) -> ()
          }
          frame #7 {
            n248 = Wait (ms)(milliseconds to wait=u32 50) -> ()  [unwired: 1 out]
          }
          frame #8 {
            n249 = local read "LimitCalc"() -> (w365:dbl)
            n250 = local read "Light"() -> (w364:dbl)
            n251 = Add(x=w365, y=w364) -> (x+y=w366:dbl)
            n252 = local write "LimitCalc"(w366) -> ()
          }
          frame #9 {
            n253 = Wait (ms)(milliseconds to wait=u32 50) -> ()  [unwired: 1 out]
          }
          frame #10 {
            n254 = local read "LimitCalc"() -> (w368:dbl)
            n255 = local read "Light"() -> (w369:dbl)
            n256 = Add(x=w368, y=w369) -> (x+y=w370:dbl)
            n257 = local write "LimitCalc"(w370) -> ()
          }
          frame #11 {
            n258 = Wait (ms)(milliseconds to wait=u32 50) -> ()  [unwired: 1 out]
          }
          frame #12 {
            n259 = local read "LimitCalc"() -> (w373:dbl)
            n260 = local read "Light"() -> (w372:dbl)
            n261 = Add(x=w373, y=w372) -> (x+y=w374:dbl)
            n262 = local write "LimitCalc"(w374) -> ()
          }
          frame #13 {
            n263 = Wait (ms)(milliseconds to wait=u32 50) -> ()  [unwired: 1 out]
          }
          frame #14 {
            n264 = local read "LimitCalc"() -> (w379:dbl)
            n265 = Divide(x=w379, y=7) -> (x/y=w376:dbl)
            "LightAvg" <- w376
            n266 = Add(x=w376, y=0.075) -> (x+y=w377:dbl)
            n267 = local write "LightLimit"(w377) -> ()
          }
        }
        n268 = Wait (ms)(milliseconds to wait=u32 10) -> ()  [unwired: 1 out]
        n269 = local read "Stop"() -> (w349:bool)
      }
      n270 = while {
        shift-right: [w650] -> _
        shift-left: _ -> [w651]
        stop <- w654 stop-if-true
        n271 = local read "Watch_Display"() -> (w653:bool)
        n272 = case shown="True" w653 {
          tunnel: w651 -> [w655 w657]
          tunnel: [w655 w656] -> w650
          frame False {
          }
          frame True {
            n273 = shared-variable "My Computer\\michelle_library.lvlib\\Display"() -> (w659:bool)  [unwired: 1 in, 1 out]
            n274 = local write "Misses"(0) -> ()
            n275 = case shown="False" w659 {
              tunnel: w657 -> [w662 w702]
              tunnel: [w660 w702] -> w656
              frame False {
                n276 = flat-sequence {
                  tunnel: w662 -> [w666]
                  tunnel: [w665] -> w661
                  tunnel: w661 -> [w692]
                  tunnel: [w691] -> w660
                  frame #0 {
                    n277 = while {
                      stop <- w681 stop-if-true
                      w682 = 10
                      n278 = local read "Its"() -> (w686:i32)
                      n279 = Wait (ms)(milliseconds to wait=w682) -> ()  [unwired: 1 out]
                      n280 = Increment(x=w686) -> (x+1=w685:i32)
                      n281 = local read "Consumption_Period"() -> (w679:i32)
                      n282 = local write "Its"(w685) -> ()
                      n283 = local read "Its"() -> (w683:i32)
                      n284 = local read "LickBurst"() -> (w687:bool)
                      n285 = Multiply(x=w683, y=w682) -> (x*y=w680:i32)
                      n286 = Greater?(x=w680, y=w679) -> (0:w678:bool)
                      n287 = Not(x=w687) -> (.not. x?=w684:bool)
                      n288 = Or(x=w684, y=w678) -> (x .or. y?=w681:bool)
                    }
                    n289 = Get Date/Time In Seconds() -> (seconds since 1Jan1904=w671:timestamp)
                    n290 = local write "Time_out"(FALSE) -> ()
                    n291 = shared-variable "My Computer\\michelle_library.lvlib\\Timeout"(FALSE) -> ()  [unwired: 1 in, 1 out]
                    n292 = local write "Active Trial"(FALSE) -> ()
                    n293 = shared-variable "My Computer\\michelle_library.lvlib\\ConsumptionON"(TRUE) -> ()  [unwired: 1 in, 1 out]
                    n294 = local read "TestTime"() -> (w668:dbl)
                    n295 = To Double Precision Float(number=w671) -> (double precision float=w669:dbl)
                    n296 = shared-variable "My Computer\\michelle_library.lvlib\\GlobalTime"() -> (w664:dbl)  [unwired: 1 in, 1 out]
                    n297 = Subtract(x=w669, y=w668) -> (x-y=w672:dbl)
                    n298 = shared-variable "My Computer\\michelle_library.lvlib\\Frame_clock"() -> (w663:u32)  [unwired: 1 in, 1 out]
                    n299 = Build Array(221, w672, w664, w663) -> (w667:T2)
                    n300 = Get Date/Time In Seconds() -> ()  [unwired: 1 out]
                    n301 = Build Array (concatenate) ("Build Matrix")(w666, w667) -> (w665:T2)
                    n302 = local write "ConsTS"(w665) -> ()
                    "ConsumptionGo" <- TRUE
                  }
                  frame #1 {
                    n303 = Get Date/Time In Seconds() -> (seconds since 1Jan1904=w696:timestamp)
                    n304 = shared-variable "My Computer\\michelle_library.lvlib\\ConsumptionON"(FALSE) -> ()  [unwired: 1 in, 1 out]
                    n305 = local write "ConsumptionGo"(FALSE ("ConsumptionGo")) -> ()
                    n306 = local write "Watch_Display"(FALSE ("Watch_Display")) -> ()
                    n307 = local read "TestTime"() -> (w693:dbl)
                    n308 = To Double Precision Float(number=w696) -> (double precision float=w694:dbl)
                    n309 = shared-variable "My Computer\\michelle_library.lvlib\\GlobalTime"() -> (w689:dbl)  [unwired: 1 in, 1 out]
                    n310 = Subtract(x=w694, y=w693) -> (x-y=w697:dbl)
                    n311 = shared-variable "My Computer\\michelle_library.lvlib\\Frame_clock"() -> (w688:u32)  [unwired: 1 in, 1 out]
                    n312 = Build Array(222, w697, w689, w688) -> (w690:T2)
                    n313 = Build Array (concatenate) ("Build Matrix")(w692, w690) -> (w691:T2)
                    n314 = local write "Its"(0) -> ()
                    n315 = local write "ConsTS"(w691) -> ()
                  }
                }
              }
              frame True {
              }
            }
          }
        }
        n316 = Wait (ms)(milliseconds to wait=u32 5) -> ()  [unwired: 1 out]
        n317 = shared-variable "My Computer\\michelle_library.lvlib\\Stop"() -> (w654:bool)  [unwired: 1 in, 1 out]
      }
      n318 = while {
        shift-right: [w385] -> _
        shift-left: _ -> [w390]
        shift-right: [w392] -> _
        shift-left: _ -> [w391]
        shift-right: [w388] -> _
        shift-left: _ -> [w387]
        stop <- w395 stop-if-true
        n319 = xnode "PhotoDiode"() -> ("C/AI0 (AI0)"=w381:dbl)  [unwired: 1 in, 1 out]
        "Light" <- w381
        n320 = Wait (ms)(milliseconds to wait=u32 1) -> ()  [unwired: 1 out]
        n321 = local read "LightLimit"() -> (w386:dbl)
        n322 = local write "LightTrig"(FALSE) -> ()
        n323 = Greater?(x=w381, y=w386) -> (0:w389:bool)
        n324 = case shown="True" w389 {
          tunnel: [w434 w436] -> w388
          tunnel: w387 -> [w434 w444]
          frame False {
          }
          frame True {
            n325 = shared-variable "My Computer\\michelle_library.lvlib\\GlobalTime"() -> (w442:dbl)  [unwired: 1 in, 1 out]
            n326 = shared-variable "My Computer\\michelle_library.lvlib\\Frame_clock"() -> (w443:u32)  [unwired: 1 in, 1 out]
            n327 = Get Date/Time In Seconds() -> (seconds since 1Jan1904=w441:timestamp)
            n328 = local read "TestTime"() -> (w439:dbl)
            n329 = To Double Precision Float(number=w441) -> (double precision float=w440:dbl)
            n330 = Subtract(x=w440, y=w439) -> (x-y=w438:dbl)
            n331 = Build Array(771, w438, w442, w443) -> (w445:T2)
            n332 = Build Array (concatenate) ("Build Matrix")(w444, w445) -> (w436:T2)
            n333 = local write "LightTS"(w436) -> ()
            "LightTrig" <- TRUE
          }
        }
        n334 = local read "LightAvg"() -> (w384:dbl)
        n335 = Subtract(x=w381, y=w384) -> (x-y=w382:dbl)
        n336 = local write "LightDeriv"(w382) -> ()
        n337 = xnode "Analog output (1 sample)"("C/AO0 (AO0)"=w381) -> ()  [unwired: 1 in, 1 out]
        n338 = Build Array (concatenate)(w391, w382) -> (w392:dbl[])
        "LightDerivPlot" <- w392
        n339 = Greater?(x=w381, y=0.5) -> (0:→"LightOn":bool)
        n340 = Build Array (concatenate)(w390, w381) -> (w385:dbl[])
        "Lightplot" <- w385
        "LightArray" <- w385
        n341 = local read "Stop"() -> (w395:bool)
      }
      n342 = flat-sequence {
        frame #0 {
          n343 = while {
            stop <- w722 stop-if-true
            n344 = shared-variable "My Computer\\michelle_library.lvlib\\Stim_loaded"() -> (w722:bool)  [unwired: 1 in, 1 out]
            "Stimuli Loaded" <- w722
          }
          n345 = Wait (ms)(milliseconds to wait=u32 10) -> ()  [unwired: 1 out]
        }
        frame #1 {
          n346 = Get Date/Time In Seconds() -> (seconds since 1Jan1904=w728:timestamp)
          n347 = local read "TestTime"() -> (w727:dbl)
          n348 = To Double Precision Float(number=w728) -> (double precision float=w726:dbl)
          n349 = shared-variable "My Computer\\michelle_library.lvlib\\InitiatedLag"() -> (w725:dbl)  [unwired: 1 in, 1 out]
          n350 = Subtract(x=w726, y=w727) -> (x-y=w723:dbl)
          n351 = Subtract(x=w723, y=w725) -> (x-y=→"Lag2":dbl)
        }
        frame #2 {
          n352 = local read "TestTime"() -> (w729:dbl)
          n353 = local read "Lag2"() -> (w730:dbl)
          n354 = Add(x=w729, y=w730) -> (x+y=w731:dbl)
          n355 = local write "TestTime"(w731) -> ()
        }
        frame #3 {
          n356 = shared-variable "My Computer\\michelle_library.lvlib\\Timings"() -> (→"Timings":dbl[])  [unwired: 1 in, 1 out]
          n357 = shared-variable "My Computer\\michelle_library.lvlib\\Stim_ID"() -> (→"Stim_ID":dbl[])  [unwired: 1 in, 1 out]
          n358 = Wait (ms)(milliseconds to wait=u32 10) -> ()  [unwired: 1 out]
          n359 = shared-variable "My Computer\\michelle_library.lvlib\\Reward_mat"() -> (→"Reward_mat":dbl[])  [unwired: 1 in, 1 out]
          n360 = shared-variable "My Computer\\michelle_library.lvlib\\Num_trials"() -> (w735:u32)  [unwired: 1 in, 1 out]
          n361 = Initialize Array(0.0 ("element"), w735) -> (→"Rewarded trials":dbl[])
        }
        frame #4 {
          n362 = while {
            shift-right: [w851] -> _
            shift-left: _ -> [w849]
            shift-right: [w847] -> _
            shift-left: _ -> [w846]
            shift-right: [w841] -> _
            shift-left: _ -> [w839]
            stop <- w852 stop-if-true
            n363 = local read "ConsumptionGo"() -> (w841:bool)
            n364 = shared-variable "My Computer\\michelle_library.lvlib\\Display"() -> (w847:bool)  [unwired: 1 in, 1 out]
            n365 = local read "Time_out"() -> (w851:bool)
            n366 = Wait (ms)(milliseconds to wait=u32 10) -> ()  [unwired: 1 out]
            n367 = Not(x=w851) -> (.not. x?=w850:bool)
            n368 = Not(x=w847) -> (.not. x?=w845:bool)
            n369 = Not(x=w841) -> (.not. x?=w842:bool)
            n370 = And(x=w850, y=w849) -> (x .and. y?=w844:bool)
            n371 = And(x=w846, y=w845) -> (x .and. y?=w840:bool)
            n372 = local read "Time_out"() -> (w848:bool)
            n373 = And(x=w839, y=w842) -> (x .and. y?=w838:bool)
            n374 = Or(x=w844, y=w840) -> (x .or. y?=w837:bool)
            n375 = Or(x=w837, y=w838) -> (x .or. y?=w836:bool)
            n376 = case shown="True" w836 {
              tunnel: w848 -> [w853 _]
              frame False {
                n377 = case shown="False" w853 {
                  frame False {
                    n378 = local read "ISI start time"() -> (w856:dbl)
                    n379 = local read "Time"() -> (w855:dbl)
                    n380 = Subtract(x=w855, y=w856) -> (x-y=w854:dbl)
                    n381 = shared-variable "My Computer\\michelle_library.lvlib\\ISI"(w854) -> ()  [unwired: 1 in, 1 out]
                    n382 = local write "ISI"(w854) -> ()
                  }
                  frame True {
                    n383 = local read "Time"() -> (w861:dbl)
                    n384 = Subtract(x=w861, y=0.11) -> (x-y=w858:dbl)
                    n385 = local write "ISI start time"(w858) -> ()
                    n386 = local read "Time"() -> (w859:dbl)
                    n387 = Subtract(x=w859, y=w858) -> (x-y=w857:dbl)
                    n388 = shared-variable "My Computer\\michelle_library.lvlib\\ISI"(w857) -> ()  [unwired: 1 in, 1 out]
                    n389 = local write "ISI"(w857) -> ()
                  }
                }
              }
              frame True {
                n390 = local read "Time"() -> (w866:dbl)
                n391 = Subtract(x=w866, y=0.11) -> (x-y=w863:dbl)
                "ISI start time" <- w863
                n392 = local read "Time"() -> (w864:dbl)
                n393 = Subtract(x=w864, y=w863) -> (x-y=w862:dbl)
                "ISI" <- w862
                n394 = shared-variable "My Computer\\michelle_library.lvlib\\ISI"(w862) -> ()  [unwired: 1 in, 1 out]
              }
            }
            n395 = local read "Stop"() -> (w852:bool)
          }
          n396 = while {
            stop <- w741 stop-if-true
            n397 = local read "Active Trial"() -> (w740:bool)
            n398 = case shown="True" w740 {
              frame False {
              }
              frame True {
                n399 = local write "Time_out"(FALSE) -> ()
                n400 = shared-variable "My Computer\\michelle_library.lvlib\\Timeout"(FALSE) -> ()  [unwired: 1 in, 1 out]
              }
            }
            n401 = Wait (ms)(milliseconds to wait=5) -> ()  [unwired: 1 out]
            n402 = shared-variable "My Computer\\michelle_library.lvlib\\Stop"() -> (w741:bool)  [unwired: 1 in, 1 out]
          }
          n403 = while {
            stop <- w762 stop-if-true
            n404 = shared-variable "My Computer\\michelle_library.lvlib\\Trial"() -> (w752:u32)  [unwired: 1 in, 1 out]
            n405 = Wait (ms)(milliseconds to wait=u32 10) -> ()  [unwired: 1 out]
            n406 = local read "Timings"() -> (w754:dbl[])
            n407 = local read "Time since lick"() -> (w761:dbl)
            n408 = Decrement(x=w752) -> (x-1=w751:u32)
            n409 = Index Array(array=w754, index=w751) -> (element=w753:dbl)
            n410 = Less?(x=w761, y=w753) -> (x < y?=w760:bool)
            n411 = shared-variable "My Computer\\michelle_library.lvlib\\Display"() -> (w757:bool)  [unwired: 1 in, 1 out]
            n412 = local read "ConsumptionGo"() -> (w749:bool)
            n413 = local read "Lick"() -> (w759:bool)
            n414 = And(x=w759, y=w760) -> (x .and. y?=w755:bool)
            n415 = Not(x=w757) -> (.not. x?=w756:bool)
            n416 = local read "Active Trial"() -> (w744:bool)
            n417 = And(x=w756, y=w755) -> (x .and. y?=w748:bool)
            n418 = Not(x=w749) -> (.not. x?=w750:bool)
            n419 = And(x=w748, y=w750) -> (x .and. y?=w746:bool)
            n420 = Not(x=w744) -> (.not. x?=w747:bool)
            n421 = And(x=w746, y=w747) -> (x .and. y?=w745:bool)
            n422 = case shown="True" w745 {
              frame False {
              }
              frame True {
                n423 = flat-sequence {
                  frame #0 {
                    w763 = TRUE
                    n424 = local read "TimeOutDuration"() -> (w764:i32)
                    n425 = xnode "DisplayOn 3"("C/DIO3 (DIO3)"=w763) -> ()  [unwired: 1 in, 1 out]
                    n426 = shared-variable "My Computer\\michelle_library.lvlib\\Timeout"(w763) -> ()  [unwired: 1 in, 1 out]
                    n427 = Wait (ms)(milliseconds to wait=w764) -> ()  [unwired: 1 out]
                    "Time_out" <- w763
                  }
                  frame #1 {
                    w800 = FALSE ("Timeout")
                    n428 = xnode "DisplayOn 4"("C/DIO3 (DIO3)"=w800) -> ()  [unwired: 1 in, 1 out]
                    n429 = local write "Time_out"(w800) -> ()
                    n430 = shared-variable "My Computer\\michelle_library.lvlib\\Timeout"(w800) -> ()  [unwired: 1 in, 1 out]
                  }
                }
              }
            }
            n431 = local read "Stop"() -> (w762:bool)
          }
          n432 = while {
            shift-right: [w913] -> _
            shift-left: _ -> [w912]
            shift-right: [w905] -> _
            shift-left: _ -> [w906]
            stop <- w915 stop-if-true
            n433 = local read "Active Trial"() -> (w910:bool)
            n434 = Wait (ms)(milliseconds to wait=u32 10) -> ()  [unwired: 1 out]
            n435 = local read "Lick"() -> (w911:bool)
            n436 = And(x=w910, y=w911) -> (x .and. y?=w909:bool)
            n437 = Or(x="Give reward", y=w909) -> (x .or. y?=w908:bool)
            n438 = case shown="True" w908 {
              tunnel: [w917 w924] -> w913
              tunnel: w912 -> [w917 w923]
              tunnel: w906 -> [w916 w921]
              tunnel: [w916 w920] -> w905
              frame False {
              }
              frame True {
                n439 = flat-sequence {
                  tunnel: w921 -> [w930]
                  tunnel: [w927] -> w918
                  tunnel: [w986] -> w919
                  tunnel: w918 -> [w984]
                  tunnel: [w1030] -> w920
                  tunnel: w919 -> [w1030]
                  frame #0 {
                    w945 = TRUE ("C/DIO0 (DIO0)")
                    n440 = Get Date/Time In Seconds() -> (seconds since 1Jan1904=w934:timestamp)
                    n441 = local write "Time_out"(FALSE) -> ()
                    n442 = shared-variable "My Computer\\michelle_library.lvlib\\Timeout"(FALSE) -> ()  [unwired: 1 in, 1 out]
                    n443 = local write "GoAhead"(FALSE) -> ()
                    n444 = Wait (ms)(milliseconds to wait=u32 100) -> ()  [unwired: 1 out]
                    n445 = local read "TestTime"() -> (w928:dbl)
                    n446 = shared-variable "My Computer\\michelle_library.lvlib\\Trial"() -> (w944:u32)  [unwired: 1 in, 1 out]
                    n447 = shared-variable "My Computer\\michelle_library.lvlib\\GlobalReward"() -> (w936:dbl)  [unwired: 1 in, 1 out]
                    n448 = To Double Precision Float(number=w934) -> (double precision float=w933:dbl)
                    n449 = shared-variable "My Computer\\michelle_library.lvlib\\GlobalTime"() -> (w926:dbl)  [unwired: 1 in, 1 out]
                    n450 = local read "Rewarded trials"() -> (w942:dbl[])
                    n451 = Subtract(x=w933, y=w928) -> (x-y=w932:dbl)
                    n452 = xnode "Reward 3"("C/DIO0 (DIO0)"=w945) -> ()  [unwired: 1 in, 1 out]
                    n453 = Decrement(x=w944) -> (x-1=w943:u32)
                    n454 = shared-variable "My Computer\\michelle_library.lvlib\\Frame_clock"() -> (w925:u32)  [unwired: 1 in, 1 out]
                    n455 = Increment(x=w936) -> (x+1=w935:dbl)
                    n456 = Replace Array Subset(array=w942, new element=1.0 ("new element/subarray"), index=w943) -> (w940:dbl[])
                    n457 = Build Array(551, w932, w926, w925) -> (w931:T2)
                    n458 = local write "Rewarded trials"(w940) -> ()
                    n459 = shared-variable "My Computer\\michelle_library.lvlib\\GlobalReward"(w935) -> ()  [unwired: 1 in, 1 out]
                    n460 = Build Array (concatenate) ("Build Matrix")(w930, w931) -> (w927:T2)
                    n461 = local write "RewTS"(w927) -> ()
                    "Reward" <- w945
                    "Watch_Display" <- w945
                  }
                  frame #1 {
                    w994 = FALSE ("C/DIO0 (DIO0)")
                    n462 = Get Date/Time In Seconds() -> (seconds since 1Jan1904=w991:timestamp)
                    n463 = local read "TestTime"() -> (w985:dbl)
                    n464 = local write "Give reward"(FALSE ("Give reward")) -> ()
                    n465 = Wait (ms)(milliseconds to wait=u32 20) -> ()  [unwired: 1 out]
                    n466 = shared-variable "My Computer\\michelle_library.lvlib\\GlobalTime"() -> (w983:dbl)  [unwired: 1 in, 1 out]
                    n467 = To Double Precision Float(number=w991) -> (double precision float=w990:dbl)
                    n468 = xnode "Reward 4"("C/DIO0 (DIO0)"=w994) -> ()  [unwired: 1 in, 1 out]
                    n469 = local write "Reward"(w994) -> ()
                    n470 = Subtract(x=w990, y=w985) -> (x-y=w989:dbl)
                    n471 = shared-variable "My Computer\\michelle_library.lvlib\\Frame_clock"() -> (w982:u32)  [unwired: 1 in, 1 out]
                    n472 = Build Array(552, w989, w983, w982) -> (w987:T2)
                    n473 = Build Array (concatenate) ("Build Matrix")(w984, w987) -> (w986:T2)
                    n474 = local write "RewTS"(w986) -> ()
                  }
                  frame #2 {
                    n475 = Wait (ms)(milliseconds to wait=u32 50) -> ()  [unwired: 1 out]
                  }
                }
                n476 = Increment(x=w923) -> (x+1=w924:u16)
                "Rewards" <- w924
                n477 = local write "Active Trial"(FALSE ("Active Trial")) -> ()
              }
            }
            n478 = local read "Stop"() -> (w915:bool)
          }
          n479 = while {
            stop <- w880 stop-if-true
            n480 = shared-variable "My Computer\\michelle_library.lvlib\\Trial"() -> (w876:u32)  [unwired: 1 in, 1 out]
            n481 = shared-variable "My Computer\\michelle_library.lvlib\\Trial"() -> (w872:u32)  [unwired: 1 in, 1 out]
            n482 = Wait (ms)(milliseconds to wait=u32 10) -> ()  [unwired: 1 out]
            n483 = local read "Rewarded trials"() -> (w873:dbl[])
            n484 = local read "Reward_mat"() -> (w875:dbl[])
            n485 = Decrement(x=w876) -> (x-1=w877:u32)
            n486 = Decrement(x=w872) -> (x-1=w871:u32)
            n487 = Index Array(array=w875, index=w877) -> (element=w878:dbl)
            n488 = Index Array(array=w873, index=w871) -> (element=w870:dbl)
            n489 = Equal To 0?(x=w870) -> (x = 0?=w869:bool)
            n490 = Equal?(x=w878, y=1.0) -> (x = y?=w868:bool)
            n491 = And(x=w868, y=w869) -> (x .and. y?=w867:bool)
            n492 = case shown="True" w867 {
              frame False {
                n493 = local write "Active Trial"(FALSE ("Active_trial")) -> ()
              }
              frame True {
                n494 = shared-variable "My Computer\\michelle_library.lvlib\\Trial"() -> (w883:u32)  [unwired: 1 in, 1 out]
                n495 = local read "Stim_ID"() -> (w885:dbl[])
                n496 = Decrement(x=w883) -> (x-1=w884:u32)
                n497 = Index Array(array=w885, index=w884) -> (element=w882:dbl)
                n498 = case shown="1, Default" w882 {
                  frame 1, Default {
                    n499 = shared-variable "My Computer\\michelle_library.lvlib\\ISI_Time"() -> (w891:dbl)  [unwired: 1 in, 1 out]
                    n500 = local read "ActiveTime"() -> (w886:dbl)
                    n501 = Less?(x=w891, y=w886) -> (x < y?=w889:bool)
                    n502 = Greater?(x=w891, y=0.1) -> (0:w888:bool)
                    n503 = And(x=w889, y=w888) -> (x .and. y?=w887:bool)
                    n504 = case shown="True" w887 {
                      frame False {
                        n505 = local write "Active Trial"(FALSE ("Active Trial")) -> ()
                      }
                      frame True {
                        n506 = local read "Time"() -> (w895:dbl)
                        n507 = local write "Active Trial"(TRUE ("Active Trial")) -> ()
                        n508 = Add(x=w895, y=-0.11) -> (x+y=w893:dbl)
                        n509 = local write "Time of last lick"(w893) -> ()
                      }
                    }
                  }
                  frame 2 {
                    n510 = shared-variable "My Computer\\michelle_library.lvlib\\ISI_Time"() -> (w901:dbl)  [unwired: 1 in, 1 out]
                    n511 = local read "ActiveTime"() -> (w897:dbl)
                    n512 = Less?(x=w901, y=w897) -> (x < y?=w899:bool)
                    n513 = Greater?(x=w901, y=0.1) -> (0:w900:bool)
                    n514 = And(x=w900, y=w899) -> (x .and. y?=w898:bool)
                    n515 = case shown="True" w898 {
                      frame False {
                        n516 = local write "Active Trial"(FALSE ("Active Trial")) -> ()
                      }
                      frame True {
                        "Active Trial" <- TRUE ("Active Trial")
                      }
                    }
                  }
                }
              }
            }
            n517 = local read "Stop"() -> (w880:bool)
          }
        }
      }
    }
  }
